vi "Creators Is Created Queue.vi"(10 "Created Queue Alias":string, 11 "eeeee in":refnum<class "eeeee.lvclass">) -> (2 "Is Created Queue?":bool, 3 "eeeee out":refnum<class "eeeee.lvclass">)   [LabVIEW 2021, in "jettl Tools.lvlib" / "eeeee.lvlib" / "eeeee.lvclass"]
uses:
  eeeee.lvclass
  eeeee.lvclass/eeeee.ctl
  jettl/Event/Event.lvclass
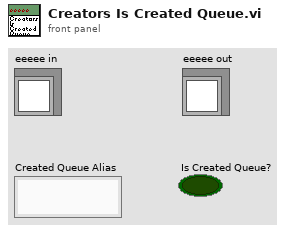
[diagram p1: front panel]
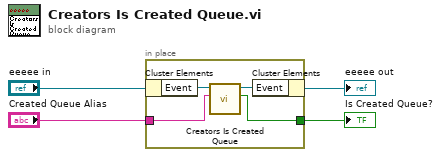
[diagram p0: block diagram]
diagram:
  n1 = in-place {
    in-place-border: "Created Queue Alias" -> [w6]
    in-place-border: [w5] -> w1
    n2 = in-place-cluster #1("eeeee in") -> ("Event"=w8:refnum<class "Event.lvclass">)
    n3 = call-dynamic "Creators Is Created Queue.vi"("Created Queue Alias"=w6, "Event in"=w8) -> ("Is Created Queue?"=w5:bool, "Event out"=w7:refnum<class "Event.lvclass">)  [unwired: 8 in]
    n4 = in-place-cluster #1("Event"=w7) -> (→"eeeee out":refnum<class "eeeee.lvclass">)
  }
  "Is Created Queue?" <- w1
